vi "Convert Code to Error.vi"(8 "error in":errorcluster, 11 "error codes":T1) -> (0 "error out":errorcluster)   [LabVIEW 2011, in "Diamond Universal Driver.lvlib"]
doc: "Convert error codes defined in the header file dscud.h to error messages based on those defined in the Error Strings section of the header file."
uses:
  Diamond Universal Driver.lvlib
  Controls/error codes.ctl
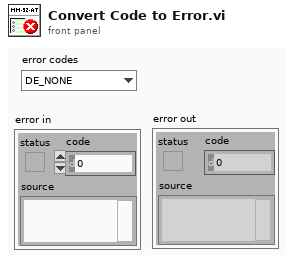
[diagram p1: front panel]
types:
  T1 = typedef "Diamond Universal Driver.lvlib/error codes.ctl" = enum8{"DE_NONE", "DE_HW_FAILURE", "DE_SW_FAILURE", "DE_HW_NOT_SUPPORTED", "DE_SW_NOT_SUPPORTED", "DE_INVALID_PARM", "DE_ALTERNATE_IN_PROGRESS", "DE_NONE_IN_PROGRESS", "DE_BUFFER_ROLLOVER", "DE_INVALID_ERROR_CODE", "DE_ALREADY_PAUSED", "DE_OVERFLOW", "DE_INVALID_FUNC", "DE_DSCUDH_INVALID", "DE_INVALID_BOARD", "DE_BOARD_LIMIT_REACHED", "DE_BOARD_BUSY", "DE_INVALID_WINDRVR_HANDLE", "DE_INVALID_WINDRVR_VERSION", "DE_BAD_WINDRVR_BOARD_INIT", "DE_OPERATION_TIMED_OUT", "DE_INVALID_WINDRVR_KP", "DE_THREAD_FAILURE"}
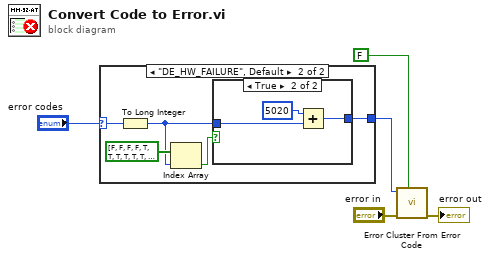
[diagram p0: block diagram]
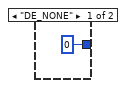
[diagram p2: hidden frame]
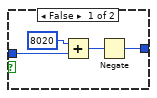
[diagram p3: hidden frame]
diagram:
  n1 = case shown="\"DE_HW_FAILURE\", Default" "error codes" {
    selector: "error codes" -> [_ w7]
    tunnel: [0 w8] -> w5
    frame "DE_NONE" {
    }
    frame "DE_HW_FAILURE", Default {
      n2 = To Long Integer(number=w7) -> (32bit integer=w9:i32)
      n3 = Index Array(array=bool[] [FALSE, FALSE, FALSE, FALSE, TRUE, TRUE, TRUE, TRUE, TRUE, TRUE, TRUE, TRUE, TRUE, FALSE, FALSE, FALSE, FALSE, FALSE, FALSE, FALSE, TRUE, FALSE, FALSE], index=w9) -> (element=w10:bool)
      n4 = case shown="True" w10 {
        tunnel: w9 -> [w14 w18]
        tunnel: [w12 w16] -> w8
        frame False {
          n5 = Add(x=8020, y=w14) -> (x+y=w13:i32)
          n6 = Negate(x=w13) -> (-x=w12:i32)
        }
        frame True {
          n7 = Add(x=5020, y=w18) -> (x+y=w16:i32)
        }
      }
    }
  }
  n8 = call <vilib>:"Error Cluster From Error Code.vi"("show call chain? (False)"=FALSE, "error in (no error)"="error in", "error code (0)"=w5) -> ("error out"=→"error out":errorcluster)  [unwired: 6 in]
